vi "test_find_surface2.vi"() -> ()   [LabVIEW 2016]
panel:
  in  "Struc El Size":i32=10
  out "Numeric":i32
  out "Array":dbl[](array[numeric])
  in  "Threshold Multiplier":sgl=2.0
  out "Num Images":dbl=1000.0
  in  "AVI File for Simulated Raw B Scan Images":path=path "C:/Users/Applied Optics Group/Desktop/DCF Paper Data Processing/data/2020_08_04_2dcheckerboard_AF/Large_grid/OCT_raw_vol.avi"
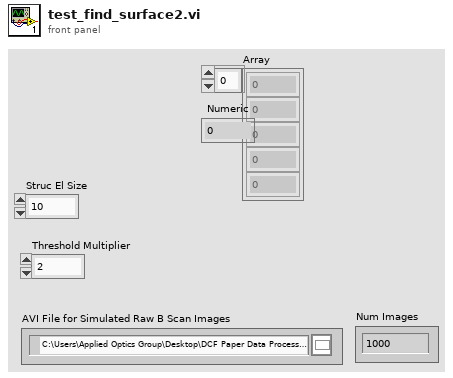
[diagram p1: front panel]
types:
  T1 = typedef "IMAQ Image.ctl" = refnum<image>
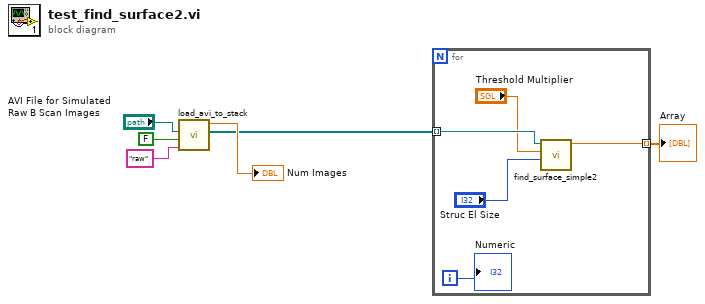
[diagram p0: block diagram]
diagram:
  n1 = call "load_avi_to_stack.vi"("Image Prefix"="raw", "Preview"=FALSE, "AVI File"="AVI File for Simulated Raw B Scan Images") -> ("Image Array"=w2:T1[], "Num Images"=→"Num Images":dbl)  [unwired: 7 in]
  n2 = for {
    tunnel: w2 -> [w11] mode=indexing
    tunnel: [w9] -> w1 mode=indexing
    i -> [w8]
    n3 = call "find_surface_simple2.vi"("Struc El Size"="Struc El Size", "Threshold Multiplier"="Threshold Multiplier", "Image In"=w11) -> ("average surface height"=w9:dbl)  [unwired: 7 in, 1 out]
    "Numeric" <- w8
  }
  "Array" <- w1
